vi "ControllingMotor_Class_P_Control_1.vi"(8 "Scale":dbl, 9 "Set Speed":dbl, 10 "Current Speed":dbl) -> (3 "New Speed":dbl)   [LabVIEW 2015]
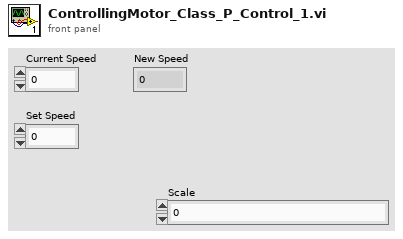
[diagram p1: front panel]
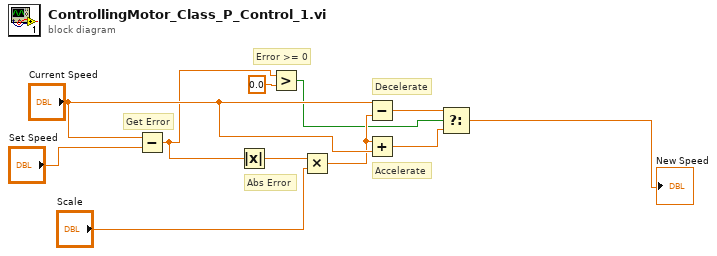
[diagram p0: block diagram]
diagram:
  # "Decelerate"
  # "Accelerate"
  # "Error >= 0"
  # "Abs Error"
  # "Get Error"
  n1 = Subtract(x="Current Speed", y="Set Speed") -> (x-y=w9:dbl)
  n2 = Absolute Value(x=w9) -> (abs(x)=w10:dbl)
  n3 = Greater?(x=w9, y=0.0) -> (0:w4:bool)
  n4 = Multiply(x=w10, y="Scale") -> (x*y=w8:dbl)
  n5 = Subtract(x="Current Speed", y=w8) -> (x-y=w7:dbl)
  n6 = Add(x=w8, y="Current Speed") -> (x+y=w6:dbl)
  n7 = Select(t=w7, s=w4, f=w6) -> (s? t:f=→"New Speed":dbl)
